vi "Release Message Queue.vi"(8 "error in (no error)":errorcluster, 11 "Message Queue":refnum<class "Message Queue.lvclass">) -> (0 "error out":errorcluster, 2 "remaining elements":refnum<class "Message.lvclass">[](array[class]))   [LabVIEW 2013, in "Actor Framework.lvlib" / "Message Queue.lvclass"]
doc: "(<B>Filename</B>: Actor Framework.lvlib:Message Queue.lvclass:Release Message Queue.vi)\n\nReleases the reference to a message queue.\n\nUse the Obtain Message Queue method to obtain the <B>Message Queue</B> input."
uses:
  <vilib>/ActorFramework/Message Queue/Message Queue.lvclass
  <vilib>/ActorFramework/Message/Message.lvclass
  <vilib>/ActorFramework/Message Queue/Message Queue.lvclass/Message Queue.ctl
  <vilib>/ActorFramework/Message Priority Queue/Message Priority Queue.lvclass
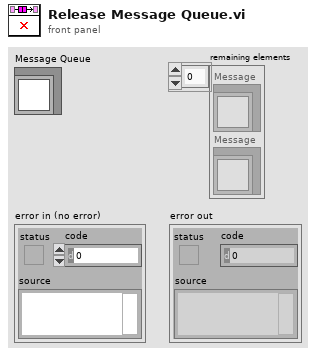
[diagram p1: front panel]
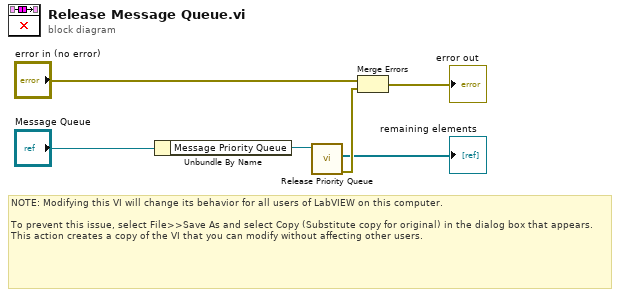
[diagram p0: block diagram]
diagram:
  # "NOTE: Modifying this VI will change its behavior for all users of LabVIEW on this computer.\n\nTo prevent this issue, select File>>Save As and select Copy (Substitute copy for original) in the dialog box that appears. This action creates a copy of the VI that you can modify without affecting other users."
  n1 = Unbundle By Name("Message Queue") -> ("Message Priority Queue"=w5:refnum<class "Message Priority Queue.lvclass">)
  n2 = call <vilib>:"Release Priority Queue.vi"("Priority Queue"=w5) -> ("error out"=w4:errorcluster, "remaining elements"=→"remaining elements":refnum<class "Message.lvclass">[])  [unwired: 9 in]
  n3 = Merge Errors("error in (no error)", w4) -> (→"error out":errorcluster)
